vi "Configure Modulation Waveform (Ramp).vi"(6 "Slope Type (0:Positive)":u16(ring) items=["Positive", "Negative"], 7 "Modulation Path (1)":u16(ring)=1 items=["1"=1, "2"=2], 8 "error in (no error)":errorcluster, 9 "Internal Source (1)":u16(ring)=1 items=["1"=1, "2"=2], 10 "Modulation Type (0: Amplitude Modulation)":u16(ring) items=["Amplitude Modulation", "Frequency Modulation", "Phase Modulation", "Low Frequency Output"], 11 "VISA resource name":refnum<visa-resource-name>) -> (0 "error out":errorcluster, 3 "VISA resource name out":refnum<visa-resource-name>)   [LabVIEW 2014, in "Agilent PSG MXG Series.lvlib"]
doc: "Configures the slope type for the ramp modulated waveform.\n\n<B>Notes:</B>\n(1) This VI is <B>NOT</B> valid in E8247C, N5161A, N5162A, N5181A, N5182A, N5183A.\n\n(2) For E8257D, E8267D, this VI is valid only when the instrument installs <B>Option UNT</B> (AM, FM, phase modulation, and LF output).\n\n(3) For N5171B, N5172B, N5181B, N5182B, this VI is valid only when the instrument installs <B>Option UNT</B> and <B>Option 303</B> (AM, FM, phase modulation, and LF output)."
uses:
  Agilent PSG MXG Series.lvlib
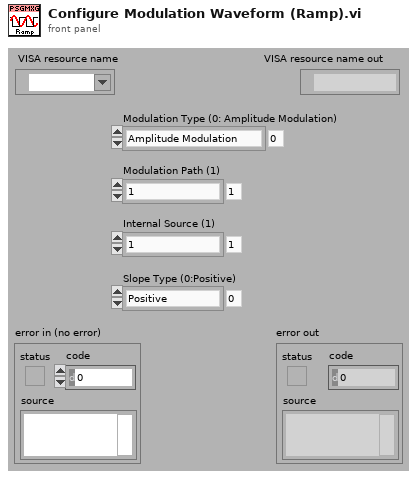
[diagram p1: front panel]
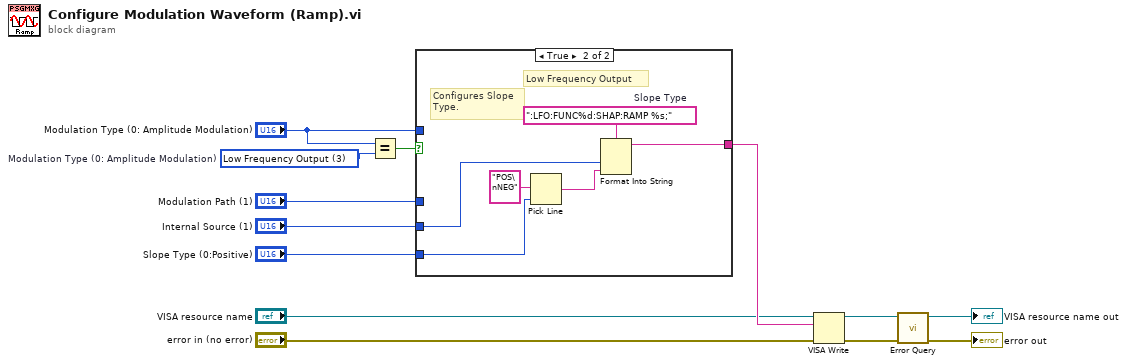
[diagram p0: block diagram]
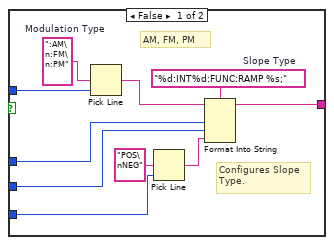
[diagram p2: hidden frame]
diagram:
  w8 = u16 3 items=["Amplitude Modulation"=0, "Frequency Modulation"=1, "Low Frequency Output"=3]  # Modulation Type (0: Amplitude Modulation)
  n1 = Equal?(x="Modulation Type (0: Amplitude Modulation)", y=w8) -> (x = y?=w13:bool)
  n2 = case shown="True" w13 {
    tunnel: "Modulation Type (0: Amplitude Modulation)" -> [w20 _]
    tunnel: "Modulation Path (1)" -> [w19 _]
    tunnel: "Internal Source (1)" -> [w18 w28]
    tunnel: "Slope Type (0:Positive)" -> [w16 w26]
    tunnel: [w14 w24] -> w12
    frame False {
      w22 = "%d:INT%d:FUNC:RAMP %s;"  # Slope Type
      w23 = ":AM\n:FM\n:PM"  # Modulation Type
      # "Configures Slope\nType."
      # "AM, FM, PM"
      n3 = Pick Line(multi-line string=w23, line index=w20) -> (output string=w21:string)  [unwired: 1 out]
      n4 = Pick Line(multi-line string="POS\nNEG", line index=w16) -> (output string=w15:string)  [unwired: 1 out]
      n5 = Format Into String(format string=w22, initial string=w21, w19, w18, w15) -> (resulting string=w14:string)  [unwired: 1 in, 1 out]
    }
    frame True {
      w29 = ":LFO:FUNC%d:SHAP:RAMP %s;"  # Slope Type
      # "Configures Slope\nType."
      # "Low Frequency Output"
      n6 = Pick Line(multi-line string="POS\nNEG", line index=w26) -> (output string=w25:string)  [unwired: 1 out]
      n7 = Format Into String(format string=w29, w28, w25) -> (resulting string=w24:string)  [unwired: 2 in, 1 out]
    }
  }
  n8 = VISA Write(VISA resource name="VISA resource name", write buffer=w12, error in (no error)="error in (no error)") -> (VISA resource name out=w11:refnum<visa-resource-name>, error out=w10:errorcluster)  [unwired: 1 out]
  n9 = call "Error Query.vi"("error in (no error)"=w10, "VISA resource name"=w11) -> ("error out"=→"error out":errorcluster, "VISA resource name out"=→"VISA resource name out":refnum<visa-resource-name>)  [unwired: 8 out]
